vi "filtra etichette NM.vi"(0 "File filtri path":path) -> (10 "all":string[](array[string]), 13 "indici grafici m,3,6":T1[](array[typedef]), 14 "Array 3ph3ch":string[](array[string]), 15 "Array 3ph6ch":string[](array[string]), 16 "Array 1ph":string[](array[string]), 17 "Filtro 3ph3ch":bool[](array[boolean]), 18 "Filtro 3ph6ch":bool[](array[boolean]), 19 "Filtro 1ph":bool[](array[boolean]))   [LabVIEW 2019]
uses:
  TypeDef/Indici.ctl
  <vilib>/Utility/file.llb/Read From Spreadsheet File (string).vi
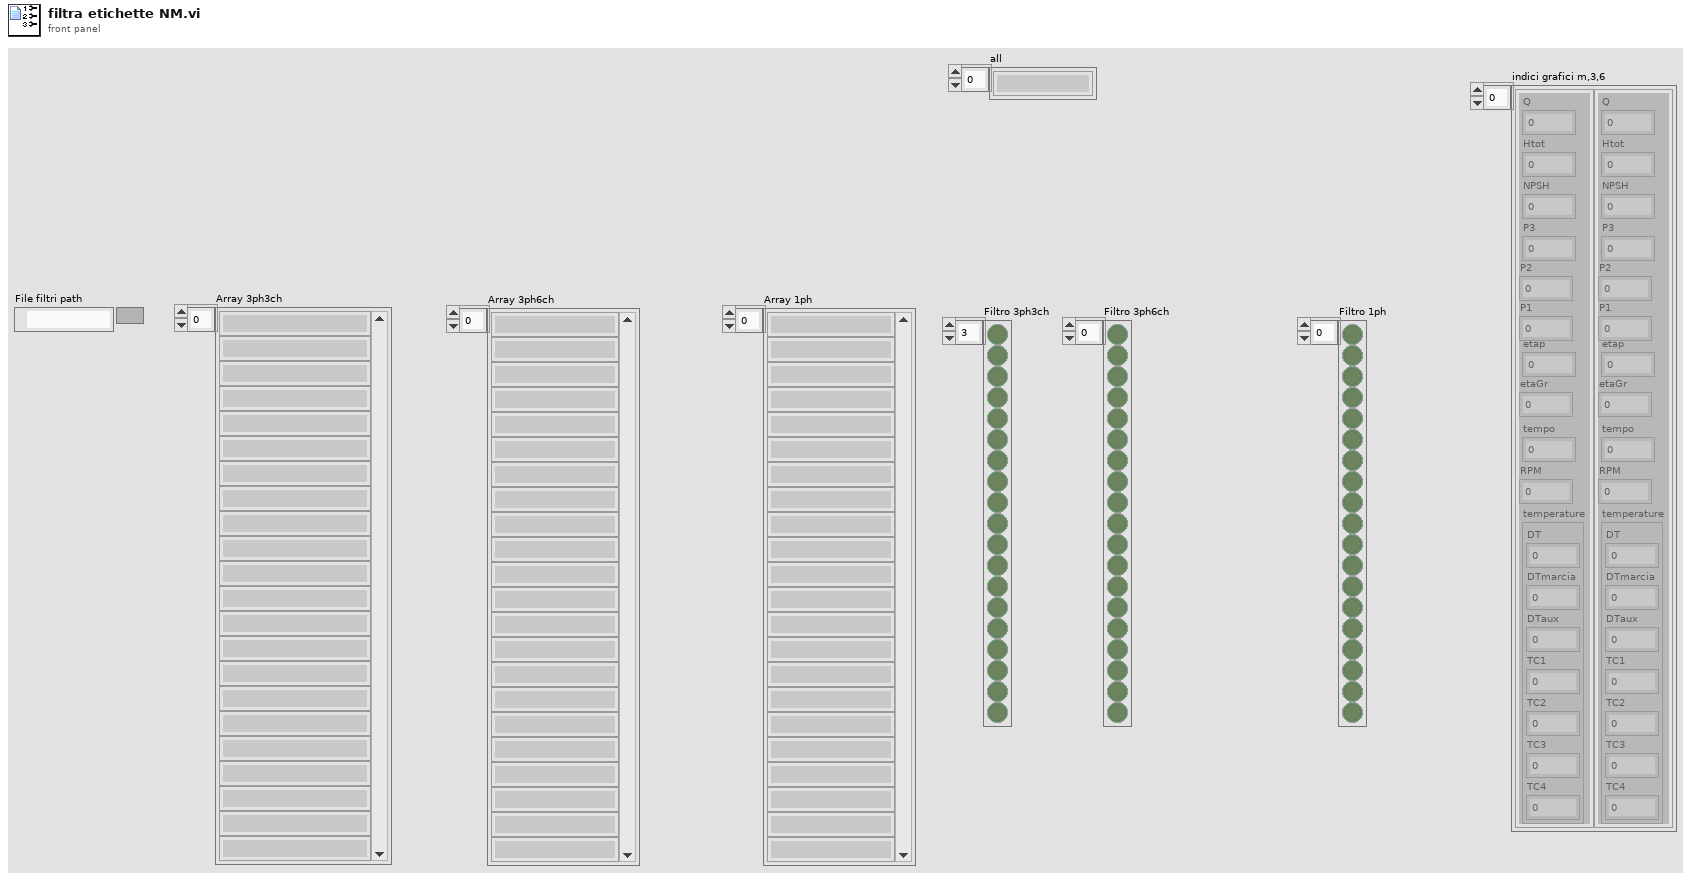
[diagram p1: front panel]
types:
  T1 = typedef "Indici.ctl" = cluster{"Q":i32, "Htot":i32, "NPSH":i32, "P3":i32, "etap":i32, "temperature":cluster{"DT":i32, "DTmarcia":i32, "DTaux":i32, "TC1":i32, "TC2":i32, "TC3":i32, "TC4":i32}, "tempo":i32, "P2":i32, "P1":i32, "etaGr":i32, "RPM":i32}
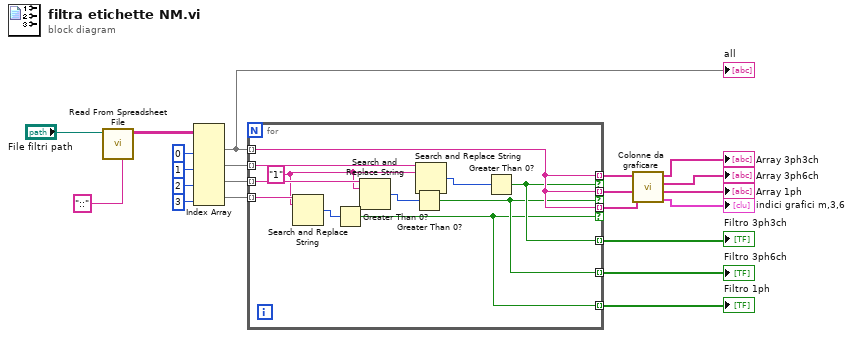
[diagram p0: block diagram]
diagram:
  n1 = call-poly <vilib>:"Read From Spreadsheet File.vi"("delimiter (\\t)"="::" ("delimiter (\\t)"), "file path (dialog if empty)"="File filtri path") -> ("all rows"=w13:string[][])  [unwired: 5 in, 4 out]
  n2 = Index Array(array=w13, index (col) #1=0 ("disabled index (col)"), index (col) #2=1 ("index (col)"), index (col) #3=2 ("index (col)"), index (col) #4=3 ("index (col)")) -> (element #1=w18:string[], element #2=w19:string[], element #3=w20:string[], element #4=w21:string[])  [unwired: 4 in]
  "all" <- w18
  n3 = for {
    tunnel: w18 -> [w32] mode=indexing
    tunnel: w19 -> [w31] mode=indexing
    tunnel: w20 -> [w29] mode=indexing
    tunnel: w21 -> [w28] mode=indexing
    tunnel: [w32] -> w7 mode=indexing if=w24
    tunnel: [w32] -> w6 mode=indexing if=w23
    tunnel: [w32] -> w5 mode=indexing if=w22
    tunnel: [w24] -> w10 mode=indexing
    tunnel: [w23] -> w9 mode=indexing
    tunnel: [w22] -> w8 mode=indexing
    w26 = "1" ("search string")
    n4 = Search and Replace String(input string=w28, search string=w26) -> (number of replacements=w27:i32)  [unwired: 6 in, 3 out]
    n5 = Greater Than 0?(x=w27) -> (x > 0?=w22:bool)
    n6 = Search and Replace String(input string=w29, search string=w26) -> (number of replacements=w25:i32)  [unwired: 6 in, 3 out]
    n7 = Greater Than 0?(x=w25) -> (x > 0?=w23:bool)
    n8 = Search and Replace String(input string=w31, search string=w26) -> (number of replacements=w30:i32)  [unwired: 6 in, 3 out]
    n9 = Greater Than 0?(x=w30) -> (x > 0?=w24:bool)
  }
  "Filtro 3ph3ch" <- w10
  "Filtro 3ph6ch" <- w9
  "Filtro 1ph" <- w8
  n10 = call "Colonne da graficare.vi"("Array 1ph"=w5, "Array 3ph6ch"=w6, "Array 3ph3ch"=w7) -> ("indici grafici m,3,6"=→"indici grafici m,3,6":T1[], "Array Array 1ph out"=→"Array 1ph":string[], "Array 3ph6ch out"=→"Array 3ph6ch":string[], "Array 3ph3ch out"=→"Array 3ph3ch":string[])  [unwired: 4 in]
